vi "Duplicate.vi"(8 "error in":errorcluster, 10 "parameters":variant, 11 "group in":refnum<class "group node.lvclass">) -> (0 "error out":errorcluster, 3 "group copy":refnum<class "group node.lvclass">)   [LabVIEW 2014, in "group node.lvclass"]
uses:
  group node.lvclass
  group node.lvclass/group node.ctl
  Read GroupName.vi
  Write GroupName.vi
  group configuration/Read groupName.vi
  group configuration/Write groupName.vi
  <vilib>/NI/Configuration Framework/serializable configuration/read metadata property.vi
  <vilib>/NI/Configuration Framework/serializable configuration/set metadata property.vi
  <vilib>/NI/Configuration Framework/serializable node/NISE_CEF_serializable node.lvclass
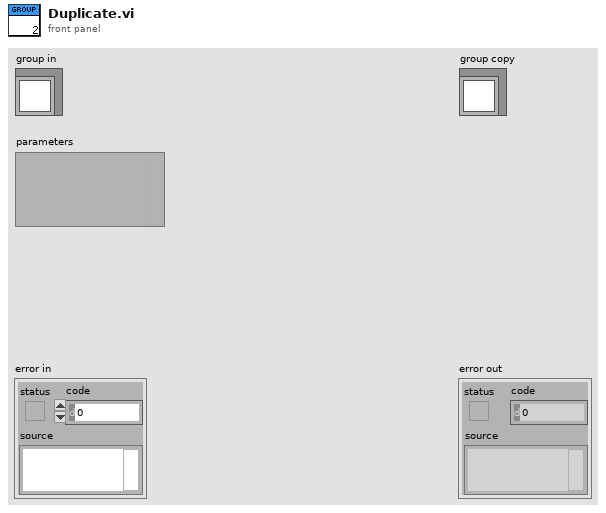
[diagram p1: front panel]
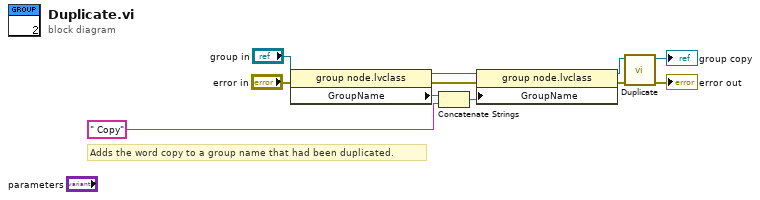
[diagram p0: block diagram]
diagram:
  # "Adds the word copy to a group name that had been duplicated."
  n1 = property class="group node.lvclass"(reference="group in", error in="error in") -> (reference out=w4:refnum<class "group node.lvclass">, error out=w7:errorcluster, "GroupName"=w2:string)
  n2 = Concatenate Strings(w2, " Copy" ("string")) -> (w1:string)
  n3 = property class="group node.lvclass"(reference=w4, error in=w7, "GroupName"=w1) -> (reference out=w3:refnum<class "group node.lvclass">, error out=w5:errorcluster)
  n4 = call-parent "Duplicate.vi"("error in"=w5, "node in"=w3) -> ("error out"=→"error out":errorcluster, "node copy out"=→"group copy":refnum<class "group node.lvclass">)  [unwired: 8 in]
